vi "Retrieve RTV [by name].vi"(0 "RT Variables in":refnum<class "RT Variables.lvclass">, 5 "RTV name":string, 11 "error in (no error)":errorcluster) -> (4 "RT Variables out":refnum<class "RT Variables.lvclass">, 6 "Data":variant, 8 "Scope":i64, 10 "RTV present?":bool, 15 "error out":errorcluster)   [LabVIEW 2019, in "LSL.lvlib" / "RT Variables.lvclass"]
uses:
  RT Variables.lvclass
  RT Variables.lvclass/RT Variables.ctl
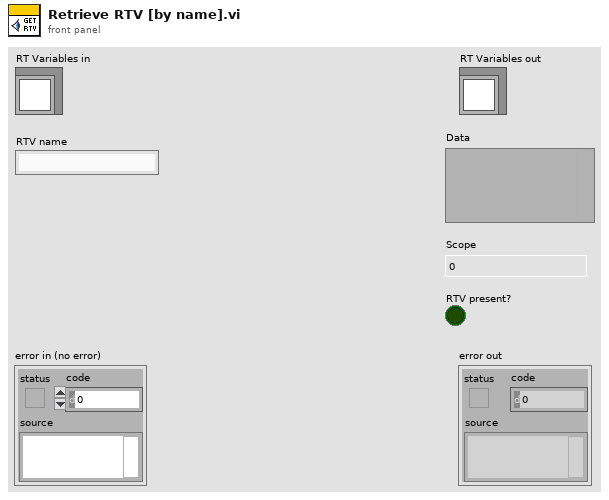
[diagram p1: front panel]
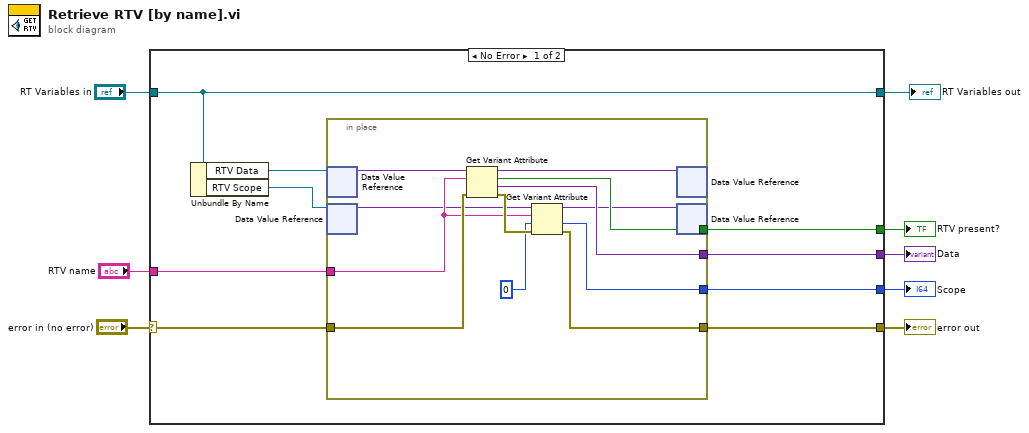
[diagram p0: block diagram]
diagram:
  n1 = case shown="No Error" "error in (no error)" {
    selector: "error in (no error)" -> [w17 w31]
    tunnel: [w16 w31] -> w7
    tunnel: "RTV name" -> [w15 _]
    tunnel: [w14 _] -> w5
    tunnel: [w13 _] -> w4
    tunnel: [w12 _] -> w3
    tunnel: "RT Variables in" -> [w9 w30]
    tunnel: [w9 w30] -> w1
    frame No Error {
      n2 = Unbundle By Name(w9) -> ("RTV Data"=w11:refnum<data-value>, "RTV Scope"=w10:refnum<data-value>)
      n3 = in-place {
        in-place-border: w17 -> [w29]
        in-place-border: [w27] -> w16
        in-place-border: w15 -> [w26]
        in-place-border: [w24] -> w14
        in-place-border: [w23] -> w13
        in-place-border: [w22] -> w12
        n4 = in-place-dvr #1(w11) -> (w21:variant)  [unwired: 1 out]
        n5 = in-place-dvr #2(w10) -> (w19:variant)  [unwired: 1 out]
        n6 = Get Variant Attribute(Variant=w21, name=w26, error in=w29) -> (duplicate Variant=w20:variant, found=w22:bool, value=w23:variant, error out=w28:errorcluster)  [unwired: 1 in]
        n7 = Get Variant Attribute(Variant=w19, name=w26, default value (empty Variant)=i64 0 ("Scope"), error in=w28) -> (duplicate Variant=w18:variant, value=w24:i64, error out=w27:errorcluster)  [unwired: 1 out]
        n8 = in-place-dvr #1(w20) -> ()  [unwired: 2 out]
        n9 = in-place-dvr #2(w18) -> ()  [unwired: 2 out]
      }
    }
    frame Error {
    }
  }
  "error out" <- w7
  "Data" <- w4
  "Scope" <- w5
  "RTV present?" <- w3
  "RT Variables out" <- w1
